vi "ReplaceLineInMultiLineString.vi"(8 "error in (no error)":errorcluster, 9 "New line":string="HVELO=30.0", 10 "Line Number":dbl, 11 "Str Refnum":refnum<vi>) -> (0 "error out":errorcluster, 3 "New string":string)   [LabVIEW 2013]
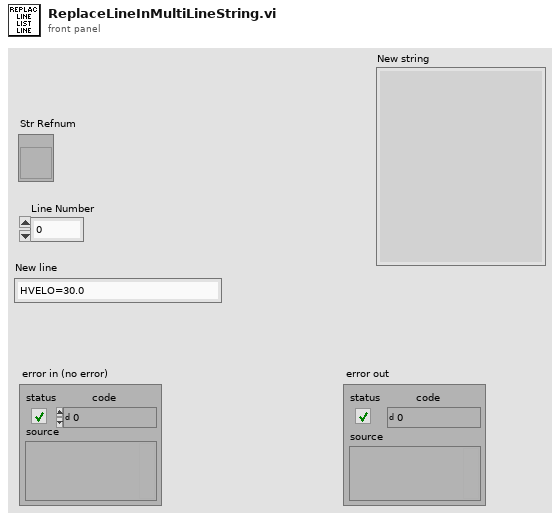
[diagram p1: front panel]
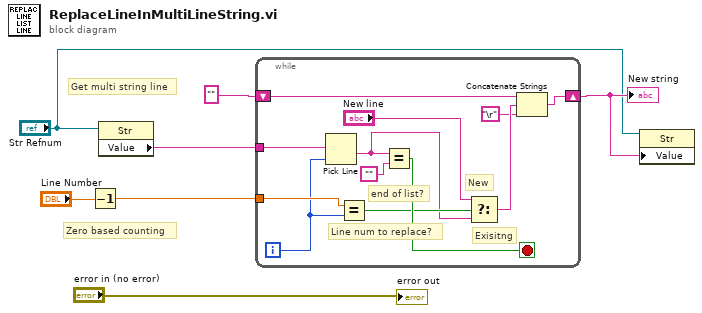
[diagram p0: block diagram]
diagram:
  # "Get multi string line"
  # "Zero based counting"
  n1 = Decrement(x="Line Number") -> (x-1=w4:dbl)
  n2 = property class="Str"(reference="Str Refnum") -> ("Value"=w6:string)  [unwired: 1 in, 2 out]
  n3 = while {
    tunnel: w6 -> [w19]
    tunnel: w4 -> [w16]
    shift-right: [w9] -> w2
    shift-left: "" -> [w11]
    i -> [w15]
    stop <- w17 stop-if-true
    # "Exisitng"
    # "New"
    # "Line num to replace?"
    # "end of list?"
    n4 = Pick Line(multi-line string=w19, line index=w15) -> (output string=w12:string)  [unwired: 1 in]
    n5 = Equal?(x=w16, y=w15) -> (x = y?=w14:bool)
    n6 = Equal?(x=w12, y="") -> (x = y?=w17:bool)
    n7 = Select(t="New line", s=w14, f=w12) -> (s? t:f=w10:string)
    n8 = Concatenate Strings(w11, w10, "\r") -> (w9:string)
  }
  "New string" <- w2
  n9 = property class="Str"(reference="Str Refnum", "Value"=w2) -> ()  [unwired: 1 in, 2 out]
  "error out" <- "error in (no error)"
